vi "Create Counter 0 Task.vi"(8 "error in":errorcluster) -> (0 "error out":errorcluster, 3 "task out":refnum<k21>)   [LabVIEW 2010, in "Core SubVIs.lvlib"]
doc: "This VI sets up an edge counting task on the 6608 (Device 1) PXI module, counter 0."
uses:
  Core SubVIs.lvlib
  <vilib>/DAQmx/create/channels.llb/DAQmx Create Channel (CI-Count Edges).vi
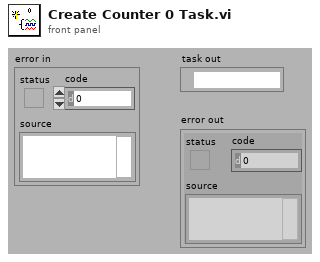
[diagram p1: front panel]
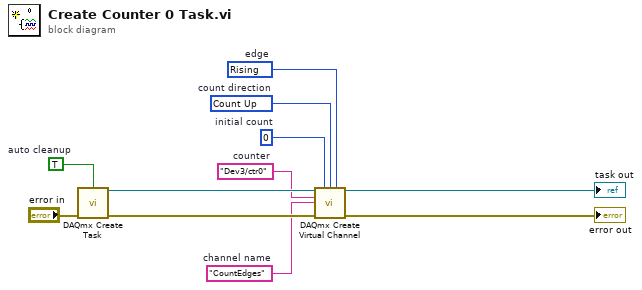
[diagram p0: block diagram]
diagram:
  w2 = 10280 items=["Rising"=10280, "Falling"=10171]  # edge
  w3 = 10128 items=["Count Up"=10128, "Count Down"=10124, "Externally Controlled"=10326]  # count direction
  w4 = u32 0  # initial count
  w5 = "CountEdges"  # channel name
  w7 = "Dev3/ctr0"  # counter
  w8 = TRUE  # auto cleanup
  n1 = call <vilib>:"DAQmx Create Task.vi"("auto cleanup"=w8, "error in"="error in") -> ("task out"=w9:refnum<k21>, "error out"=w10:errorcluster)  [unwired: 3 in, 9 out]
  n2 = call-poly <vilib>:"DAQmx Create Virtual Channel.vi"("task in"=w9, "initial count"=w4, "count direction"=w3, "edge"=w2, "counter"=w7, "name to assign"=w5, "error in"=w10) -> ("task out"=→"task out":refnum<k21>, "error out"=→"error out":errorcluster)  [unwired: 7 out]
